vi "New TDMS Sink.vi"(8 "error in (no error)":errorcluster, 10 "Group Name":string, 11 "TDMS File Path":path) -> (0 "error out":errorcluster, 3 "TDMS out":refnum<class "TDMS Sink.lvclass">)   [LabVIEW 2020, in "LV Log.lvlib" / "TDMS Sink.lvclass"]
uses:
  TDMS Sink.lvclass
  TDMS Sink.lvclass/TDMS Sink.ctl
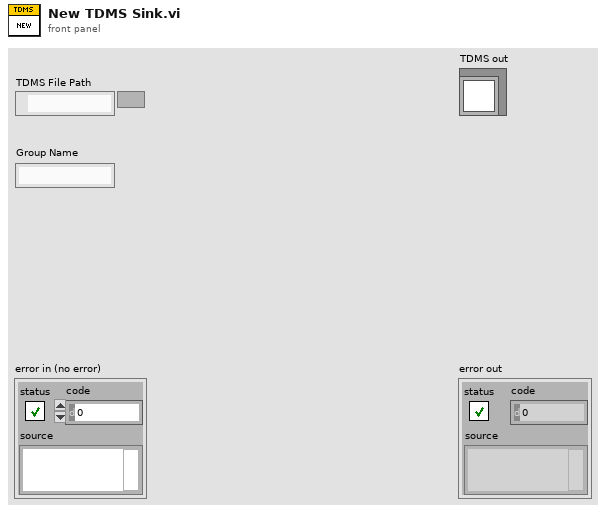
[diagram p1: front panel]
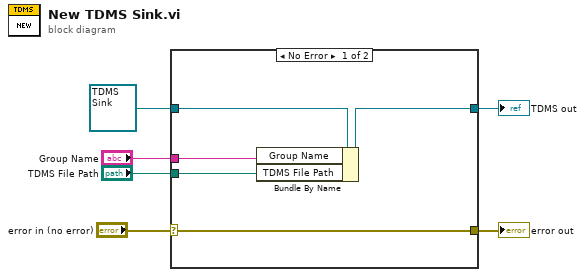
[diagram p0: block diagram]
diagram:
  n1 = case shown="No Error" "error in (no error)" {
    selector: "error in (no error)" -> [w9 w13]
    tunnel: [w9 w13] -> w5
    tunnel: [w10 w12] -> w3
    tunnel: refnum<class "TDMS Sink.lvclass"> refnum ("TDMS in") -> [w11 w12]
    tunnel: "TDMS File Path" -> [w8 _]
    tunnel: "Group Name" -> [w7 _]
    frame No Error {
      n2 = Bundle By Name(cluster=w11, "Group Name"=w7, "TDMS File Path"=w8) -> (w10:refnum<class "TDMS Sink.lvclass">)
    }
    frame Error {
    }
  }
  "error out" <- w5
  "TDMS out" <- w3
